vi "Test Get FeedbackNode Loop Init Terminal.vi"() -> ()   [LabVIEW 2014]
panel:
  out "Array":string[](array[string])
  in  "vi path":path
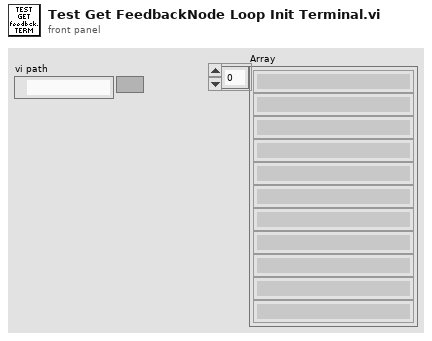
[diagram p1: front panel]
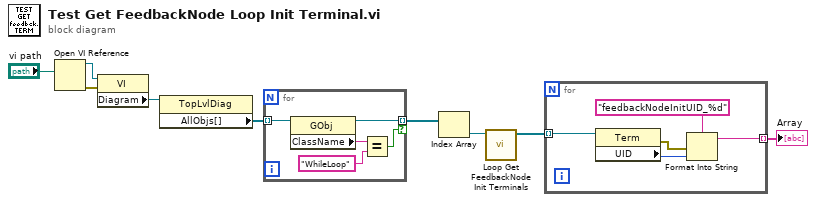
[diagram p0: block diagram]
diagram:
  n1 = Open VI Reference(vi path="vi path") -> (vi reference=w8:refnum<vi>, error out=w7:errorcluster)  [unwired: 5 in]
  n2 = property class="VI"(reference=w8, error in=w7) -> ("Diagram"=w6:refnum<vi>)  [unwired: 2 out]
  n3 = property class="TopLvlDiag"(reference=w6) -> ("AllObjs[]"=w5:refnum<vi>[])  [unwired: 1 in, 2 out]
  n4 = for {
    tunnel: w5 -> [w14] mode=indexing
    tunnel: [w11] -> w4 mode=indexing if=w10
    n5 = property class="GObj"(reference=w14) -> (reference out=w11:refnum<vi>, "ClassName"=w13:string)  [unwired: 1 in, 1 out]
    n6 = Equal?(x=w13, y="WhileLoop") -> (x = y?=w10:bool)
  }
  n7 = Index Array(array=w4) -> (element=w3:refnum<vi>)  [unwired: 1 in]
  n8 = call "Loop Get FeedbackNode Init Terminals.vi"("GObject in"=w3) -> ("feedback nodes init terms[]"=w2:refnum<vi>[])  [unwired: 10 in]
  n9 = for {
    tunnel: w2 -> [w19] mode=indexing
    tunnel: [w15] -> w1 mode=indexing
    n10 = property class="Term"(reference=w19) -> (error out=w18:errorcluster, "UID"=w17:i32)  [unwired: 1 in, 1 out]
    n11 = Format Into String(format string="feedbackNodeInitUID_%d", error in=w18, w17) -> (resulting string=w15:string)  [unwired: 1 in, 1 out]
  }
  "Array" <- w1
